vi "Material-Line 2-Normalize.vi"(8 "error in (no error)":errorcluster, 11 "Material-RunTest in":refnum<class "Material-RunTest.lvclass">) -> (0 "error out":errorcluster, 3 "Material-RunTest out":refnum<class "Material-RunTest.lvclass">)   [LabVIEW 2013, in "Material-RunTest.lvclass"]
uses:
  Material-RunTest.lvclass
  Material-RunTest.lvclass/Material-RunTest.ctl
  <userlib>/_MGI/1D Array/MGI Average/MGI Average (DBL[]).vi
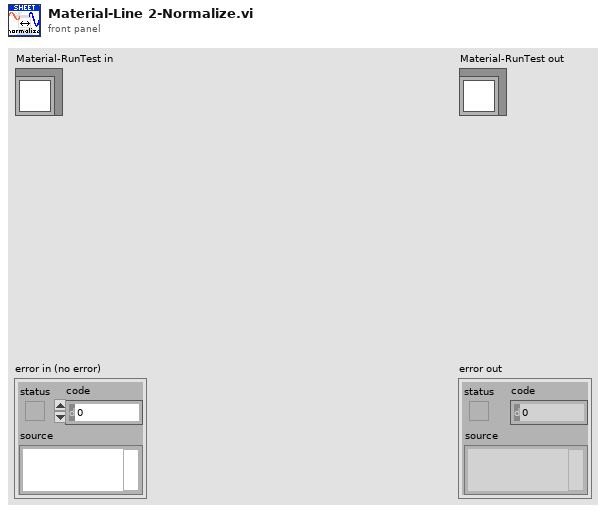
[diagram p1: front panel]
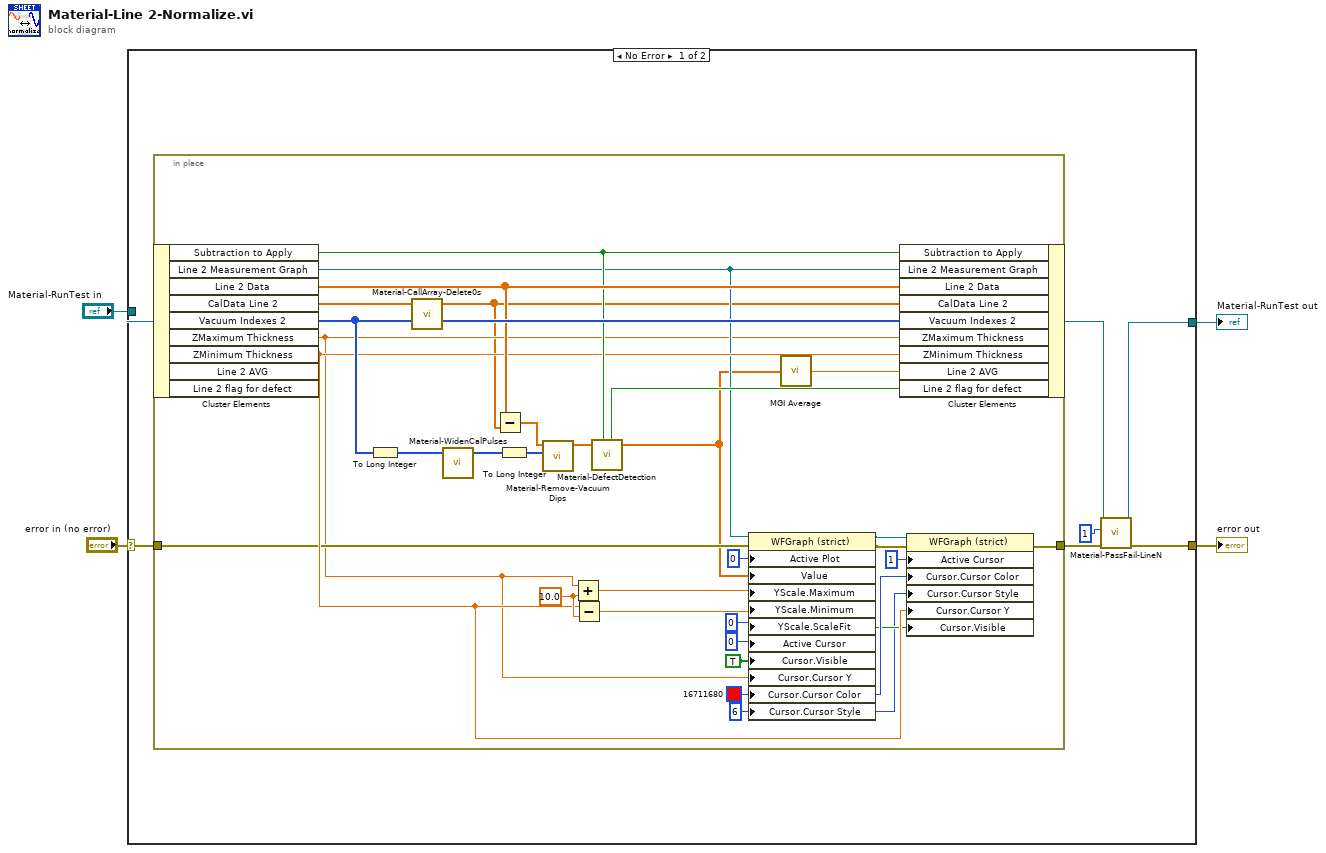
[diagram p0: block diagram]
diagram:
  n1 = case shown="No Error" "error in (no error)" {
    selector: "error in (no error)" -> [w10 w43]
    tunnel: [w7 w43] -> w3
    tunnel: [w5 w42] -> w1
    tunnel: "Material-RunTest in" -> [w11 w42]
    frame No Error {
      n2 = in-place {
        in-place-border: w10 -> [w27]
        in-place-border: [w32] -> w9
        w16 = u32 16711680
        w14 = u8 6 ("Cursor.Cursor Style")
        w15 = TRUE ("Cursor.Visible")
        w37 = 10.0 ("y")
        n3 = in-place-cluster #1(w11) -> ("Subtraction to Apply"=w30:bool, "Line 2 Measurement Graph"=w26:refnum<vi>, "Line 2 Data"=w35:dbl[], "CalData Line 2"=w13:dbl[], "Vacuum Indexes 2"=w36:i32[], "ZMaximum Thickness"=w23:dbl, "ZMinimum Thickness"=w28:dbl)  [unwired: 2 out]
        n4 = To Long Integer(number=w36) -> (32bit integer=w38:i32[])
        n5 = call "Material-CallArray-Delete0s.vi"("CalData Line 3"=w13) -> ("array w/ subset deleted"=w12:dbl[])  [unwired: 8 in]
        n6 = call "Material-WidenCalPulses.vi"("raw CAL indexes"=w38) -> ("New Indexes"=w40:u32[])  [unwired: 8 in]
        n7 = Subtract(x=w35, y=w12) -> (x-y=w39:dbl[])
        n8 = To Long Integer(number=w40) -> (32bit integer=w41:i32[])
        n9 = call "Material-Remove-VacuumDips.vi"("input array of indexes"=w41, "Input Data"=w39) -> ("Conditioned output"=w31:dbl[])  [unwired: 9 in]
        n10 = Add(x=w23, y=w37) -> (x+y=w21:dbl)
        n11 = Subtract(x=w28, y=w37) -> (x-y=w20:dbl)
        n12 = call "Material-DefectDetection.vi"("Conditioned output"=w31, "Subtraction to Apply"=w30) -> ("Flagged for Defect"=w29:bool, "Array"=w22:dbl[])  [unwired: 6 in]
        n13 = property class="WFGraph (strict)"(reference=w26, error in=w27, "Active Plot"=u32 0, "Value"=w22, "YScale.Maximum"=w21, "YScale.Minimum"=w20, "YScale.ScaleFit"=u8 0 ("Y Scale.Scale Fit"), "Active Cursor"=u32 0, "Cursor.Visible"=w15, "Cursor.Cursor Y"=w23, "Cursor.Cursor Color"=w16, "Cursor.Cursor Style"=w14) -> (reference out=w25:refnum<vi>, error out=w24:errorcluster)
        n14 = call-poly <userlib>:"MGI Average.vi"("Double[]"=w22) -> ("Average"=w34:dbl)  [unwired: 1 in]
        n15 = in-place-cluster #1("Subtraction to Apply"=w30, "Line 2 Measurement Graph"=w26, "Line 2 Data"=w35, "CalData Line 2"=w12, "Vacuum Indexes 2"=w36, "ZMaximum Thickness"=w23, "ZMinimum Thickness"=w28, "Line 2 AVG"=w34, "Line 2 flag for defect"=w29) -> (w6:refnum<class "Material-RunTest.lvclass">)
        n16 = property class="WFGraph (strict)"(reference=w25, error in=w24, "Active Cursor"=u32 1, "Cursor.Cursor Color"=w16, "Cursor.Cursor Style"=w14, "Cursor.Cursor Y"=w28, "Cursor.Visible"=w15) -> (error out=w32:errorcluster)  [unwired: 1 out]
      }
      n17 = call "Material-PassFail-LineN.vi"("error in (no error)"=w9, "Line?"=1, "Material-RunTest in"=w6) -> ("error out"=w7:errorcluster, "Material-RunTest out"=w5:refnum<class "Material-RunTest.lvclass">)  [unwired: 7 in]
    }
    frame Error {
    }
  }
  "error out" <- w3
  "Material-RunTest out" <- w1
